vi "Set SeperatedLayers.vi"(7 "OutputDirPath":path, 8 "error in (no error)":errorcluster, 9 "Sorted Heads[]":u8[](array[numeric]), 10 "Images":T1[](array[typedef]), 11 "DLP2 in":refnum<class "DLP2.lvclass">) -> (0 "error out":errorcluster, 3 "DLP2 out":refnum<class "DLP2.lvclass">)   [LabVIEW 2022 SP3, in "DLP2.lvclass"]
doc: "Developed by Kevin Thompson\nkevin@thompsonengineering.net\n\nCopyright 2018\nThompson Engineering, LLC"
uses:
  DLP2.lvclass
  DLP2.lvclass/DLP2.ctl
  <vilib>/vision/Image Controls.llb/IMAQ Image.ctl
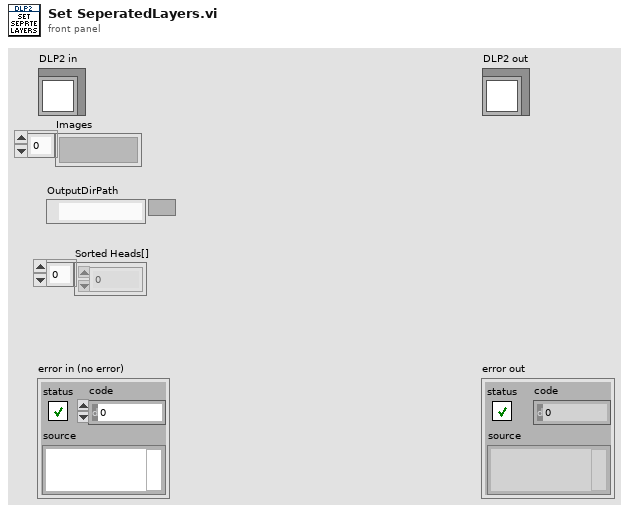
[diagram p1: front panel]
types:
  T1 = typedef "IMAQ Image.ctl" = refnum<image>
  T2 = typedef "DLP2.lvclass/ObjData--cluster.ctl" = cluster{"Settings":T3, "Public Events":T4, "Dependency":T5, "ReadData-placeholder":T6, "VISA-placeholder":refnum<visa-resource-name>, "Images":T1[], "Sorted Heads[]":u8[]}
  T3 = typedef "DLP2.lvclass/Settings--cluster.ctl" = cluster{"Simulation":bool}
  T4 = typedef "DLP2.lvclass/Public Events--cluster.ctl" = cluster{"Temp01.AsyncCmd Event":refnum<user-event>, "Temp01.AsyncMsg Event":refnum<user-event>, "stop process":refnum<user-event>, "API Incoming Event":refnum<user-event>, "API Executed Event":refnum<user-event>, "API Return Event":refnum<user-event>, "Images":refnum<user-event>}
  T5 = typedef "DLP2.lvclass/Dependency--cluster.ctl" = cluster{"Config":refnum<class>, "Database":refnum<class "Database.lvclass">}
  T6 = typedef "DLP2.lvclass/Read Data--cluster.ctl" = cluster{"Data":dbl}
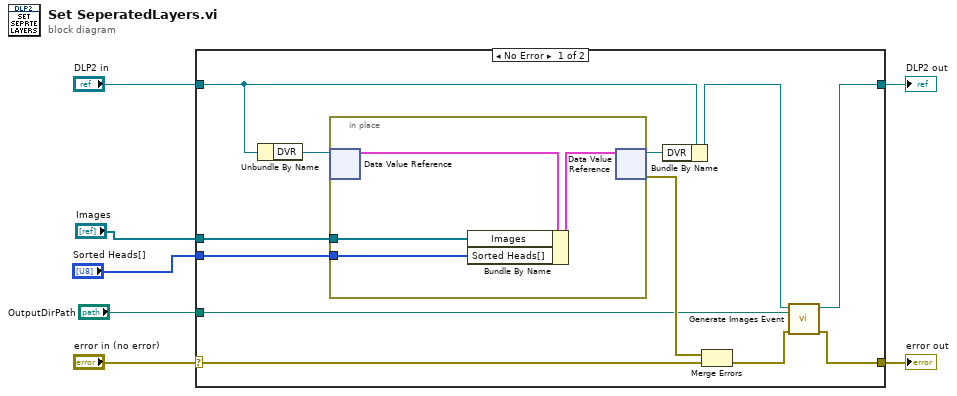
[diagram p0: block diagram]
diagram:
  n1 = case shown="No Error" "error in (no error)" {
    selector: "error in (no error)" -> [w19 w24]
    tunnel: [w10 w24] -> w6
    tunnel: [w12 w25] -> w4
    tunnel: "DLP2 in" -> [w18 w25]
    tunnel: "Images" -> [w14 _]
    tunnel: "OutputDirPath" -> [w9 _]
    tunnel: "Sorted Heads[]" -> [w8 _]
    frame No Error {
      n2 = Unbundle By Name(w18) -> ("DVR"=w17:refnum<data-value>)
      n3 = in-place {
        in-place-border: w14 -> [w21]
        in-place-border: w8 -> [w20]
        n4 = in-place-dvr #1(w17) -> (w23:T2)  [unwired: 1 out]
        n5 = Bundle By Name(cluster=w23, "Images"=w21, "Sorted Heads[]"=w20) -> (w22:T2)
        n6 = in-place-dvr #1(w22) -> (w16:refnum<data-value>, w15:errorcluster)
      }
      n7 = Bundle By Name(cluster=w18, "DVR"=w16) -> (w13:refnum<class "DLP2.lvclass">)
      n8 = Merge Errors(w15, w19) -> (w11:errorcluster)
      n9 = call "Generate Images Event.vi"("error in (no error)"=w11, "OutputDirPath"=w9, "DLP2 in"=w13) -> ("error out"=w10:errorcluster, "DLP2 out"=w12:refnum<class "DLP2.lvclass">)  [unwired: 7 in]
    }
    frame Error {
    }
  }
  "error out" <- w6
  "DLP2 out" <- w4
